vi "PPMS.Get All.vi"(8 "error in (no error)":errorcluster, 11 "instrument.PPMS in":refnum<class "instrument.PPMS.lvclass">) -> (0 "error out":errorcluster, 2 "getAll":T1, 3 "instrument.PPMS out":refnum<class "instrument.PPMS.lvclass">)   [LabVIEW 2019, in "instrument.PPMS.lvclass"]
uses:
  instrument.PPMS.lvclass
  Typedefs/PPMS.getAll--cluster.ctl
  instrument.PPMS.lvclass/instrument.PPMS.ctl
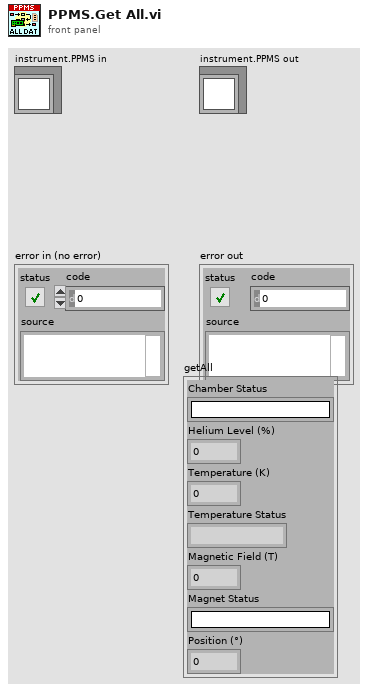
[diagram p1: front panel]
types:
  T1 = typedef "instrument.PPMS.lvclass/PPMS.getAll--cluster.ctl" = cluster{"Chamber Status":string, "Helium Level (%)":dbl, "Temperature (K)":dbl, "Temperature Status":string, "Magnetic Field (T)":dbl, "Magnet Status":string, "Position (°)":dbl}
  T2 = typedef "instrument.PPMS.lvclass/PPMS.Temperature Status--cluster.ctl" = cluster{"Temperature (K)":dbl, "Temperature Status":string}
  T3 = typedef "instrument.PPMS.lvclass/PPMS.Magnet Status--cluster.ctl" = cluster{"Field (T)":dbl, "Magnet Status":string}
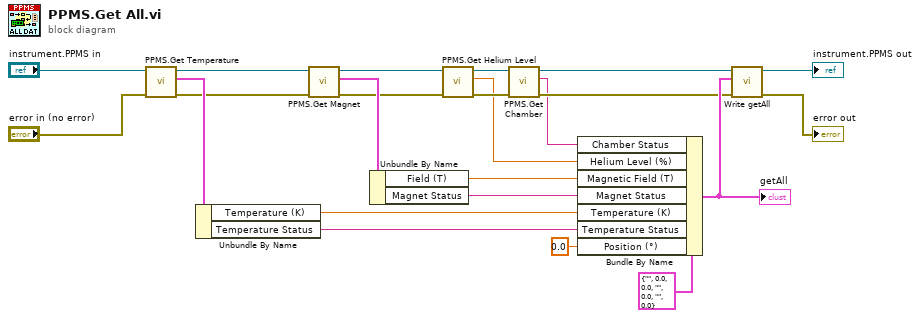
[diagram p0: block diagram]
diagram:
  n1 = call "PPMS.Get Temperature.vi"("error in (no error)"="error in (no error)", "instrument.PPMS"="instrument.PPMS in") -> ("error out"=w3:errorcluster, "Temperature Status"=w12:T2, "instrument.PPMS out"=w1:refnum<class "instrument.PPMS.lvclass">)  [unwired: 7 in]
  n2 = Unbundle By Name(w12) -> ("Temperature (K)"=w5:dbl, "Temperature Status"=w6:string)
  n3 = call "PPMS.Get Magnet.vi"("error in (no error)"=w3, "instrument.PPMS"=w1) -> ("error out"=w4:errorcluster, "Magnet Status"=w13:T3, "instrument.PPMS out"=w2:refnum<class "instrument.PPMS.lvclass">)  [unwired: 7 in]
  n4 = Unbundle By Name(w13) -> ("Field (T)"=w8:dbl, "Magnet Status"=w7:string)
  n5 = call "PPMS.Get Helium Level.vi"("error in (no error)"=w4, "instrument.PPMS"=w2) -> ("error out"=w15:errorcluster, "Helium Level (%)"=w9:dbl, "instrument.PPMS out"=w14:refnum<class "instrument.PPMS.lvclass">)  [unwired: 7 in]
  n6 = call "PPMS.Get Chamber.vi"("error in (no error)"=w15, "instrument.PPMS"=w14) -> ("error out"=w21:errorcluster, "Status String"=w16:string, "instrument.PPMS out"=w18:refnum<class "instrument.PPMS.lvclass">)  [unwired: 7 in]
  n7 = Bundle By Name(cluster=T1 {"Chamber Status"="", "Helium Level (%)"=0.0, "Temperature (K)"=0.0, "Temperature Status"="", "Magnetic Field (T)"=0.0, "Magnet Status"="", "Position (°)"=0.0} ("getAll"), "Chamber Status"=w16, "Helium Level (%)"=w9, "Magnetic Field (T)"=w8, "Magnet Status"=w7, "Temperature (K)"=w5, "Temperature Status"=w6, "Position (°)"=0.0) -> (w23:T1)
  "getAll" <- w23
  n8 = call "Write getAll.vi"("error in (no error)"=w21, "getAll"=w23, "instrument.PPMS in"=w18) -> ("error out"=→"error out":errorcluster, "instrument.PPMS out"=→"instrument.PPMS out":refnum<class "instrument.PPMS.lvclass">)  [unwired: 7 in]
